vi "UploadCalibrDataFromTXT.vi"(5 "Enable":bool, 7 "error in":errorcluster, 9 "Cluster in":T1, 10 "VISA Refnum in":refnum<visa-resource-name>) -> (0 "error out":errorcluster, 1 "transposed array":i64[][](array[numeric]))   [LabVIEW 2020]
uses:
  <vilib>/Utility/file.llb/Read From Spreadsheet File (I64).vi
panel:
  in  "file path (dialog if empty)":path
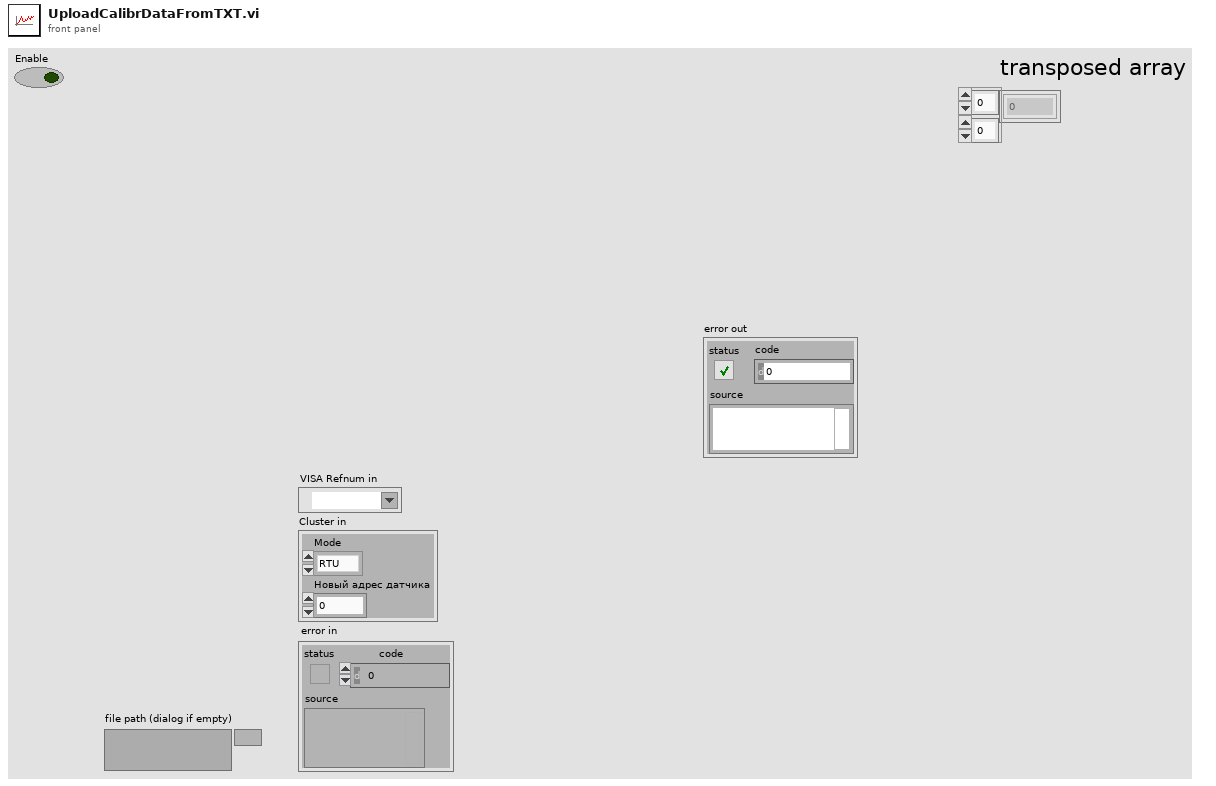
[diagram p1: front panel]
types:
  T1 = cluster{"Mode":enum16{"RTU", "ASCII"}, "Новый адрес датчика":u16}
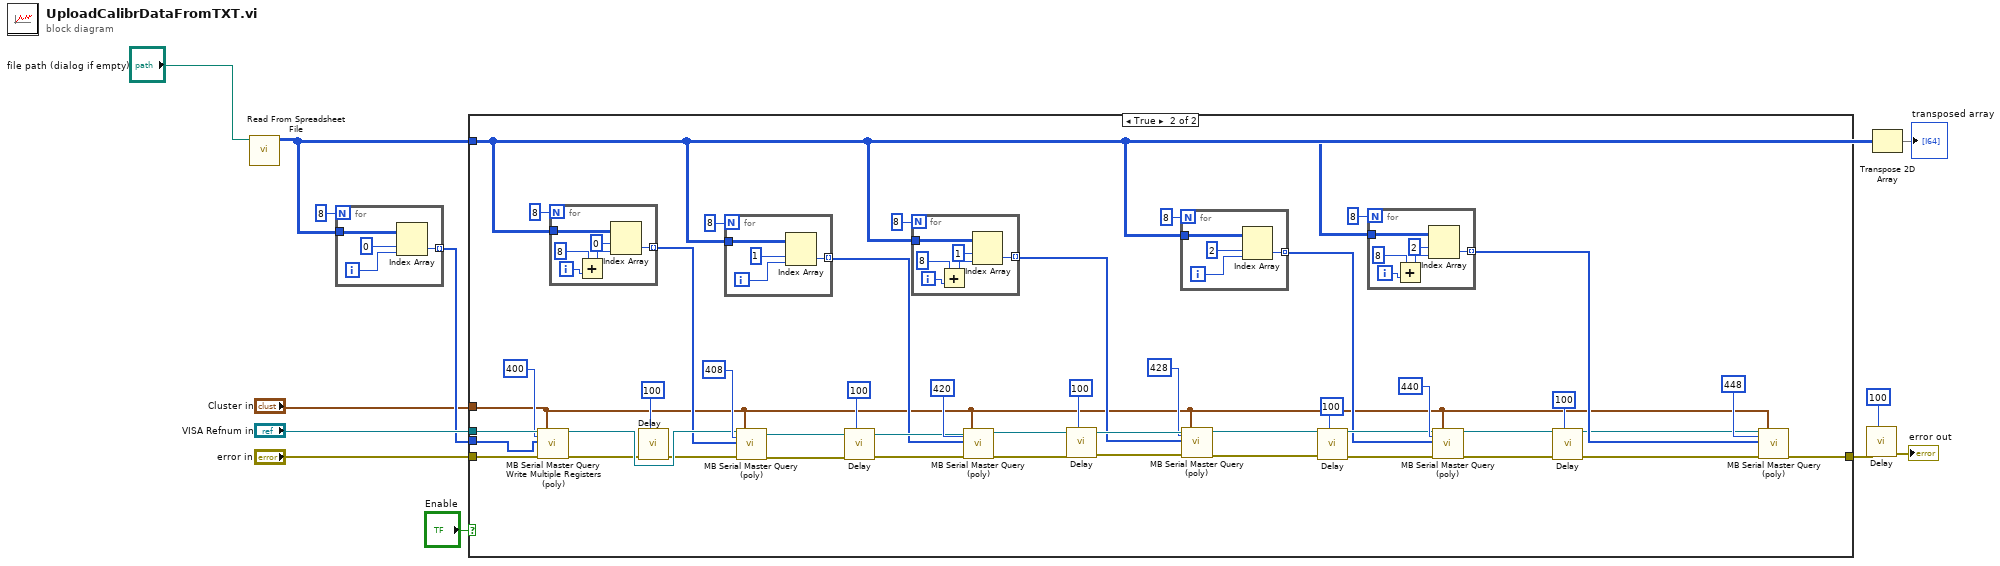
[diagram p0: block diagram]
diagram:
  n1 = call-poly <vilib>:"Read From Spreadsheet File.vi"("file path (dialog if empty)"="file path (dialog if empty)") -> ("all rows"=w3:i64[][])  [unwired: 6 in, 4 out]
  n2 = for {
    N: 8 -> [_]
    tunnel: w3 -> [w16]
    tunnel: [w13] -> w9 mode=indexing
    i -> [w14]
    n3 = Index Array(array=w16, index (row)=0, index (col)=w14) -> (element=w13:i64)
  }
  n4 = case shown="True" "Enable" {
    tunnel: "VISA Refnum in" -> [_ w59]
    tunnel: "error in" -> [w17 w58]
    tunnel: w9 -> [_ w18]
    tunnel: "Cluster in" -> [_ w22]
    tunnel: [w17 w20] -> w6
    tunnel: w3 -> [_ w19]
    frame False {
    }
    frame True {
      n5 = call <vilib>:"MB Serial Master Query Write Multiple Registers (poly).vi"("VISA resource name"=w59, "Starting Address"=u16 400 ("Command"), "Registers"=w18, "error in"=w58, "Serial Parameters"=w22) -> ("VISA resource name out"=w51:refnum<visa-resource-name>, "error out"=w50:errorcluster)  [unwired: 12 in, 1 out]
      n6 = for {
        N: 8 -> [_]
        tunnel: [w85] -> w35 mode=indexing
        tunnel: w19 -> [w82]
        i -> [w84]
        n7 = Add(x=8, y=w84) -> (x+y=w81:i32)
        n8 = Index Array(array=w82, index (row)=0 ("disabled index (row)"), index (col)=w81) -> (element=w85:i64)
      }
      n9 = call "Delay.vi"("milliseconds to wait"=u32 100, "error in (no error)"=w50) -> ("error out"=w49:errorcluster)  [unwired: 8 in, 1 out]
      n10 = for {
        N: 8 -> [_]
        tunnel: w19 -> [w79]
        tunnel: [w76] -> w38 mode=indexing
        i -> [w77]
        n11 = Index Array(array=w79, index (row)=1, index (col)=w77) -> (element=w76:i64)
      }
      n12 = call-poly <vilib>:"MB Serial Master Query (poly).vi"("VISA resource name"=w51, "Starting Address"=u16 408 ("Command"), "Registers"=w35, "error in"=w49, "Serial Parameters"=w22) -> ("VISA resource name out"=w45:refnum<visa-resource-name>, "error out"=w44:errorcluster)  [unwired: 1 in, 12 out]
      n13 = call "Delay.vi"("milliseconds to wait"=u32 100, "error in (no error)"=w44) -> ("error out"=w43:errorcluster)  [unwired: 8 in, 1 out]
      n14 = for {
        N: 8 -> [_]
        tunnel: [w75] -> w37 mode=indexing
        tunnel: w19 -> [w72]
        i -> [w74]
        n15 = Add(x=8, y=w74) -> (x+y=w71:i32)
        n16 = Index Array(array=w72, index (row)=1 ("disabled index (row)"), index (col)=w71) -> (element=w75:i64)
      }
      n17 = call-poly <vilib>:"MB Serial Master Query (poly).vi"("VISA resource name"=w45, "Starting Address"=u16 420 ("Command"), "Registers"=w38, "error in"=w43, "Serial Parameters"=w22) -> ("VISA resource name out"=w42:refnum<visa-resource-name>, "error out"=w41:errorcluster)  [unwired: 1 in, 12 out]
      n18 = call "Delay.vi"("milliseconds to wait"=u32 100, "error in (no error)"=w41) -> ("error out"=w47:errorcluster)  [unwired: 8 in, 1 out]
      n19 = for {
        N: 8 -> [_]
        tunnel: w19 -> [w69]
        tunnel: [w66] -> w24 mode=indexing
        i -> [w67]
        n20 = Index Array(array=w69, index (row)=2, index (col)=w67) -> (element=w66:i64)
      }
      n21 = call-poly <vilib>:"MB Serial Master Query (poly).vi"("VISA resource name"=w42, "Starting Address"=u16 428 ("Command"), "Registers"=w37, "error in"=w47, "Serial Parameters"=w22) -> ("VISA resource name out"=w31:refnum<visa-resource-name>, "error out"=w30:errorcluster)  [unwired: 1 in, 12 out]
      n22 = call "Delay.vi"("milliseconds to wait"=u32 100, "error in (no error)"=w30) -> ("error out"=w33:errorcluster)  [unwired: 8 in, 1 out]
      n23 = for {
        N: 8 -> [_]
        tunnel: [w65] -> w23 mode=indexing
        tunnel: w19 -> [w62]
        i -> [w64]
        n24 = Add(x=8, y=w64) -> (x+y=w61:i32)
        n25 = Index Array(array=w62, index (row)=2 ("disabled index (row)"), index (col)=w61) -> (element=w65:i64)
      }
      n26 = call-poly <vilib>:"MB Serial Master Query (poly).vi"("VISA resource name"=w31, "Starting Address"=u16 440 ("Command"), "Registers"=w24, "error in"=w33, "Serial Parameters"=w22) -> ("VISA resource name out"=w21:refnum<visa-resource-name>, "error out"=w28:errorcluster)  [unwired: 1 in, 12 out]
      n27 = call "Delay.vi"("milliseconds to wait"=u32 100, "error in (no error)"=w28) -> ("error out"=w27:errorcluster)  [unwired: 8 in, 1 out]
      n28 = call-poly <vilib>:"MB Serial Master Query (poly).vi"("VISA resource name"=w21, "Starting Address"=u16 448 ("Command"), "Registers"=w23, "error in"=w27, "Serial Parameters"=w22) -> ("error out"=w20:errorcluster)  [unwired: 1 in, 13 out]
    }
  }
  n29 = call "Delay.vi"("milliseconds to wait"=u32 100, "error in (no error)"=w6) -> ("error out"=→"error out":errorcluster)  [unwired: 8 in, 1 out]
  n30 = Transpose 2D Array(2D array=w3) -> (transposed array=→"transposed array":i64[][])
